vi "read data.vi"(8 "error in (no error)":errorcluster, 11 "Thermocouples in":refnum<class "Thermocouples.lvclass">) -> (0 "error out":errorcluster, 2 "data":dbl format="%0.2f", 3 "Thermocouples out":refnum<class "Thermocouples.lvclass">)   [LabVIEW 2025, in "Thermocouples.lvclass"]
uses:
  Thermocouples.lvclass
  Thermocouples.lvclass/Thermocouples.ctl
  <vilib>/DAQmx/read.llb/DAQmx Read (Analog DBL 1Chan 1Samp).vi
  <vilib>/DAQmx/miscellaneous.llb/DAQmx Fill In Error Info.vi
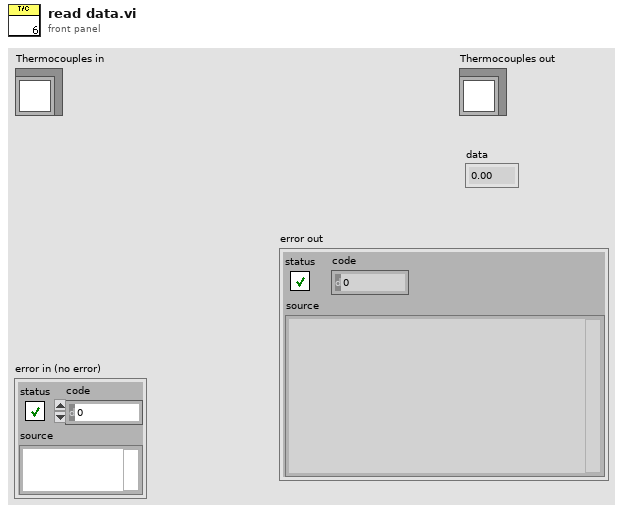
[diagram p1: front panel]
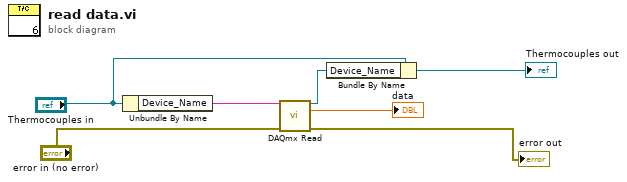
[diagram p0: block diagram]
diagram:
  n1 = Unbundle By Name("Thermocouples in") -> ("Device_Name"=w7:string)
  n2 = call-poly <vilib>:"DAQmx Read.vi"("task/channels in"=w7, "error in"="error in (no error)") -> ("task out"=w3:refnum<k21>, "data"=→"data":dbl, "error out"=→"error out":errorcluster)  [unwired: 11 in]
  n3 = Bundle By Name(cluster="Thermocouples in", "Device_Name"=w3) -> (→"Thermocouples out":refnum<class "Thermocouples.lvclass">)
